vi "DSF.Engine.BuilderManager.Wait for Builder Response.vi"(8 "error in (no error)":errorcluster, 9 "expected response":T1, 10 "Builder":refnum<class "DSF.Engine.Builder.lvclass">, 11 "Builder Manager in":refnum<class "DSF.Engine.BuilderManager.lvclass">) -> (0 "error out":errorcluster, 3 "Builder Manager out":refnum<class "DSF.Engine.BuilderManager.lvclass">)   [LabVIEW 2017, in "DSF.Engine.lvlib" / "DSF.Engine.BuilderManager.lvclass"]
uses:
  DSF.Engine.BuilderManager.lvclass
  Builder/DSF.Engine.Builder.lvclass
  Interface/DSF.Engine.Interface.Builder.Response Data.ctl
  Interface/DSF.Engine.Interface.Builder.Response.ctl
  Builder/DSF.Engine.Builder.lvclass/DSF.Engine.Builder.ctl
  Interface/DSF.Engine.Interface.Builder.Read.Response.vi
  Interface/DSF.Engine.Interface.Builder.lvclass
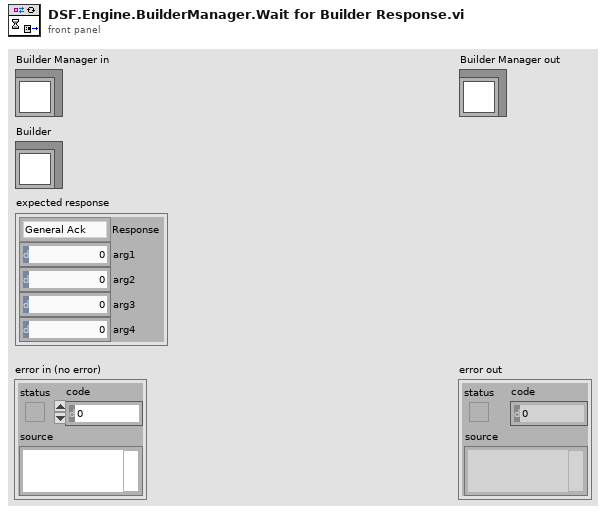
[diagram p1: front panel]
types:
  T1 = typedef "DSF.Engine.lvlib/DSF.Engine.Interface.Builder.lvclass/DSF.Engine.Interface.Builder.Response Data.ctl" = cluster{"Response":T2, "arg1":i32, "arg2":i32, "arg3":i32, "arg4":i32}
  T2 = typedef "DSF.Engine.lvlib/DSF.Engine.Interface.Builder.lvclass/DSF.Engine.Interface.Builder.Response.ctl" = enum8{"General Ack", "Initialize Complete", "Build Complete", "Parse Complete", "Shutdown Ack"}
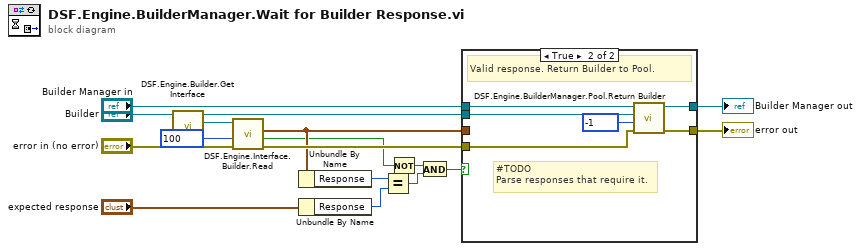
[diagram p0: block diagram]
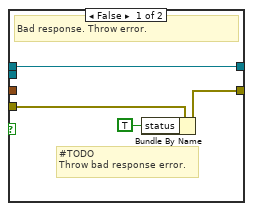
[diagram p2: hidden frame]
diagram:
  n1 = call "DSF.Engine.Builder.Get Interface.vi"("Builder in"="Builder") -> ("Builder Interface"=w16:refnum<class "DSF.Engine.Interface.Builder.lvclass">, "Builder out"=w10:refnum<class "DSF.Engine.Builder.lvclass">)  [unwired: 9 in]
  n2 = call-poly "DSF.Engine.Interface.Builder.Read.vi"("error in (no error)"="error in (no error)", "timeout in ms (0)"=100, "Builder Interface in"=w16) -> ("error out"=w4:errorcluster, "empty?"=w1:bool, "response"=w2:T1)  [unwired: 4 in, 2 out]
  n3 = Unbundle By Name(w2) -> ("Response"=w14:T2)
  n4 = Unbundle By Name("expected response") -> ("Response"=w13:T2)
  n5 = Equal?(x=w14, y=w13) -> (x = y?=w6:bool)
  n6 = Not(x=w1) -> (.not. x?=w3:bool)
  n7 = And(x=w3, y=w6) -> (x .and. y?=w11:bool)
  n8 = case shown="True" w11 {
    tunnel: w2 -> [_ _]
    tunnel: w10 -> [_ w23]
    tunnel: "Builder Manager in" -> [w21 w27]
    tunnel: [w21 w26] -> w8
    tunnel: [w19 w25] -> w7
    tunnel: w4 -> [w20 w22]
    frame False {
      # "#TODO\nThrow bad response error."
      # "Bad response. Throw error."
      n9 = Bundle By Name(cluster=w20, "status"=TRUE) -> (w19:errorcluster)
    }
    frame True {
      # "#TODO\nParse responses that require it."
      # "Valid response. Return Builder to Pool."
      n10 = call "DSF.Engine.BuilderManager.Pool.Return Builder.vi"("error in (no error)"=w22, "timeout in ms"=-1, "Builder"=w23, "Builder Manager in"=w27) -> ("error out"=w25:errorcluster, "Builder Manager out"=w26:refnum<class "DSF.Engine.BuilderManager.lvclass">)  [unwired: 5 in, 1 out]
    }
  }
  "error out" <- w7
  "Builder Manager out" <- w8
